vi "Obtain Serial Session.vi"(7 "Session Name ()":string="Serial Session", 8 "error in":errorcluster, 11 "Serial Session in":refnum<class "Serial Session.lvclass">) -> (0 "error out":errorcluster, 2 "created new?":bool, 3 "hSerial":T1)   [LabVIEW 2015, in "Serial Session.lvclass"]
doc: "Obtain a new handle for a serial session."
uses:
  Serial Session.lvclass
  Typedefs/Session Handle.ctl
  _Session Fwk/Session - Root.lvclass
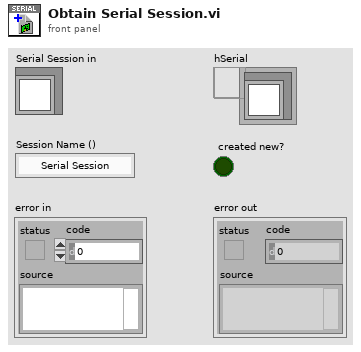
[diagram p1: front panel]
types:
  T1 = typedef "Serial Session.lvclass/Session Handle.ctl" = refnum<data-value>
  T2 = typedef "Session - Root.lvclass/Session Handle.ctl" = refnum<data-value>
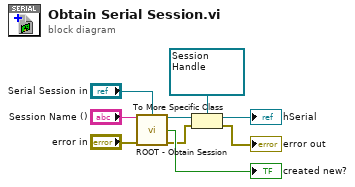
[diagram p0: block diagram]
diagram:
  n1 = call "ROOT - Obtain Session.vi"("Session Name ()"="Session Name ()", "OBJ - Session"="Serial Session in", "error in (no error)"="error in") -> ("Session Handle"=w6:T2, "created new?"=→"created new?":bool, "error out"=w5:errorcluster)  [unwired: 10 in]
  n2 = To More Specific Class(target class=T1 refnum ("Session Handle"), reference=w6, error in=w5) -> (specific class reference=→"hSerial":T1, error out=→"error out":errorcluster)
